vi "connect test.vi"() -> ()   [LabVIEW 2026]
panel:
  out "Response":string
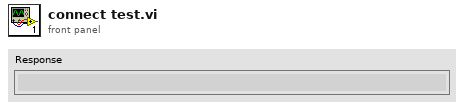
[diagram p1: front panel]
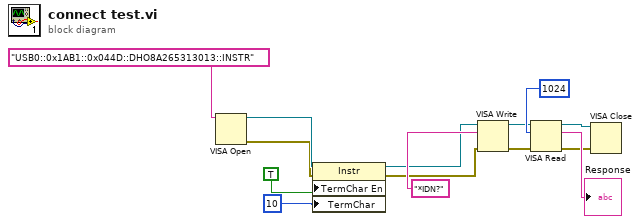
[diagram p0: block diagram]
diagram:
  n1 = VISA Open(VISA resource name="USB0::0x1AB1::0x044D::DHO8A265313013::INSTR") -> (VISA resource name=w4:refnum<visa-resource-name>, error out=w3:errorcluster)  [unwired: 4 in]
  n2 = property class="Instr"(reference=w4, error in=w3, "TermChar En"=TRUE, "TermChar"=10) -> (reference out=w1:refnum<visa-resource-name>, error out=w2:errorcluster)
  n3 = VISA Write(VISA resource name=w1, write buffer="*IDN?", error in (no error)=w2) -> (VISA resource name out=w13:refnum<visa-resource-name>, error out=w10:errorcluster)  [unwired: 1 out]
  n4 = VISA Read(VISA resource name=w13, byte count=1024, error in (no error)=w10) -> (VISA resource name out=w12:refnum<visa-resource-name>, read buffer=→"Response":string, error out=w9:errorcluster)  [unwired: 1 out]
  n5 = VISA Close(VISA resource name=w12, error in (no error)=w9) -> ()  [unwired: 1 out]
